vi "CTRE_Phoenix_CANcoder_SetCustomParameter.vi"(0 "CTRE_CANcoder_DeviceRef":T1, 5 "paramIdx":u32, 7 "value":i32, 11 "error in":errorcluster, 12 "timeoutMs":i32) -> (4 "CTRE_CANcoder_DeviceRef":T1, 15 "error out":errorcluster)   [LabVIEW 2020]
doc: "Sets the custom parameter value."
uses:
  <vilib>/Rock Robotics/WPI/ThirdParty/Phoenix-LabVIEW/CANCoder/Controls/CTRE_Phoenix_CANcoder_DeviceRef.ctl
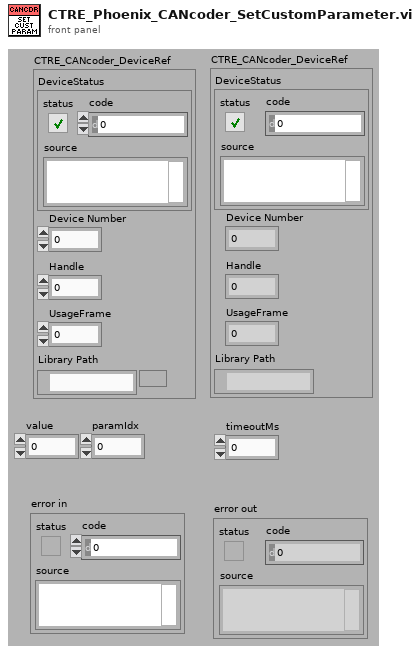
[diagram p1: front panel]
types:
  T1 = typedef "CTRE_Phoenix_CANcoder_DeviceRef.ctl" = cluster{"DeviceStatus":errorcluster, "Device Number":u8, "Handle":u64, "UsageFrame":u32, "Library Path":path}
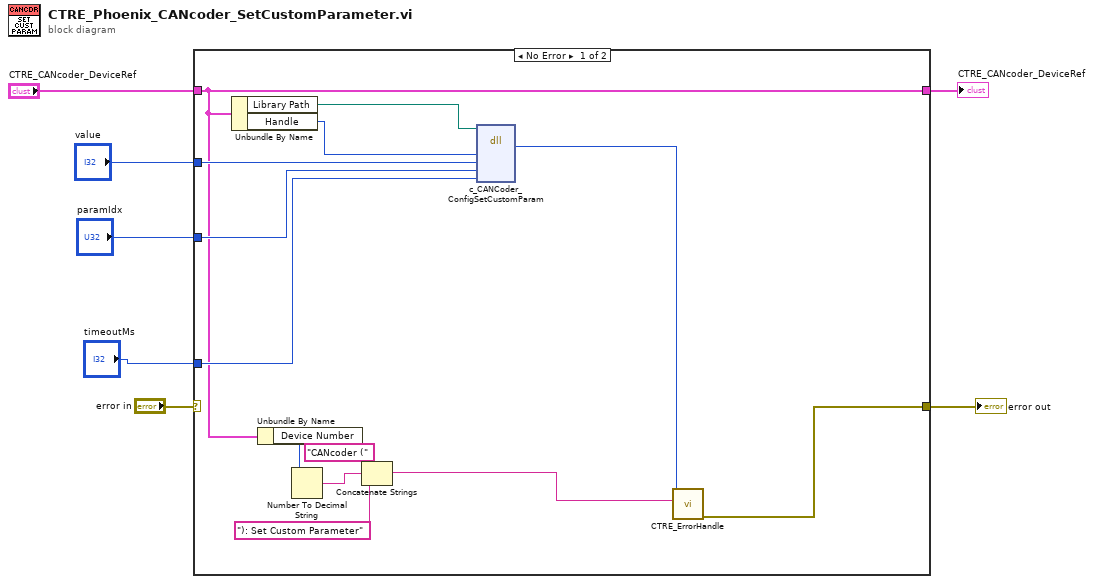
[diagram p0: block diagram]
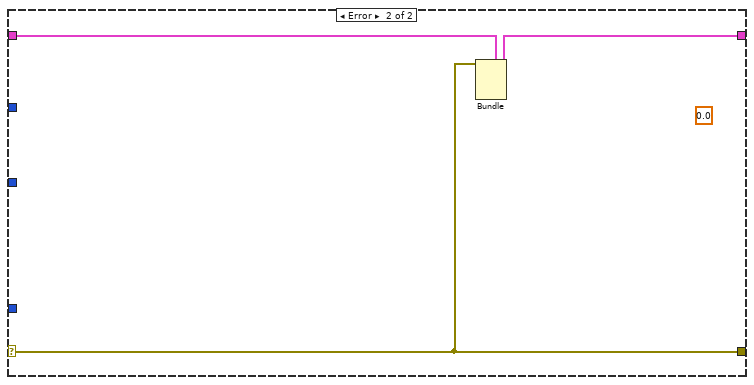
[diagram p2: hidden frame]
diagram:
  n1 = case shown="No Error" "error in" {
    selector: "error in" -> [_ w22]
    tunnel: "CTRE_CANcoder_DeviceRef" -> [w10 w23]
    tunnel: [w20 w22] -> w7
    tunnel: [w10 w21] -> w1
    tunnel: "timeoutMs" -> [w13 _]
    tunnel: "value" -> [w12 _]
    tunnel: "paramIdx" -> [w11 _]
    frame No Error {
      n2 = Unbundle By Name(w10) -> ("Library Path"=w9:path, "Handle"=w8:u64)
      n3 = Unbundle By Name(w10) -> ("Device Number"=w16:u8)
      n4 = Number To Decimal String(number=w16) -> (decimal integer string=w18:string)  [unwired: 1 in]
      n5 = Concatenate Strings("CANcoder (" ("string"), w18, "): Set Custom Parameter" ("string")) -> (w14:string)
      n6 = dll-call lib="?" fn="c_CANCoder_ConfigSetCustomParam"(path in=w9, "handle"=w8, "newValue"=w12, "paramIdx"=w11, "timeoutMs"=w13) -> ("return type"=w15:i32)  [unwired: 6 in, 2 out]
      n7 = call <vilib>:"CTRE_ErrorHandle.vi"("origin"=w14, "code"=w15) -> ("error out"=w20:errorcluster)  [unwired: 9 in]
    }
    frame Error {
      (unwired) sgl 0.0 ("value")
      n8 = Bundle(cluster=w23, "DeviceStatus"=w22) -> (w21:T1)  [unwired: 4 in]
    }
  }
  "error out" <- w7
  "CTRE_CANcoder_DeviceRef" <- w1
